vi "__List Drag Start Handler.vi"(8 "error in (no error)":errorcluster, 11 "MCListbox Refnum":refnum<vi>) -> (0 "error out":errorcluster, 2 "Discard Drag?":bool, 3 "Drag Data":T1(array[cluster]))   [LabVIEW 2011]
doc: "This VI decides if the drag operation is discarded on start (if the selected item is not a file in one of the listboxes).\nIn case the operation is allowed, it also created the necessary drag data."
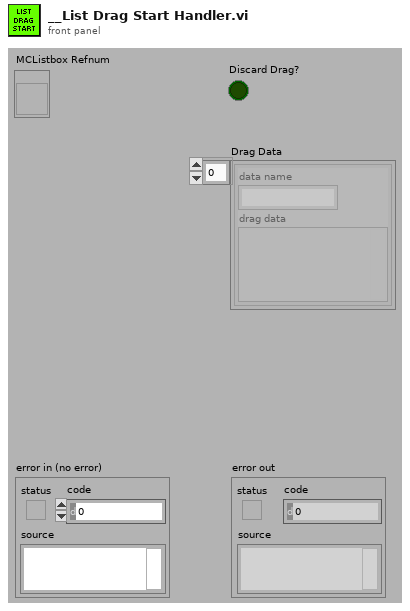
[diagram p1: front panel]
types:
  T1 = cluster{"data name":string, "drag data":variant}[]
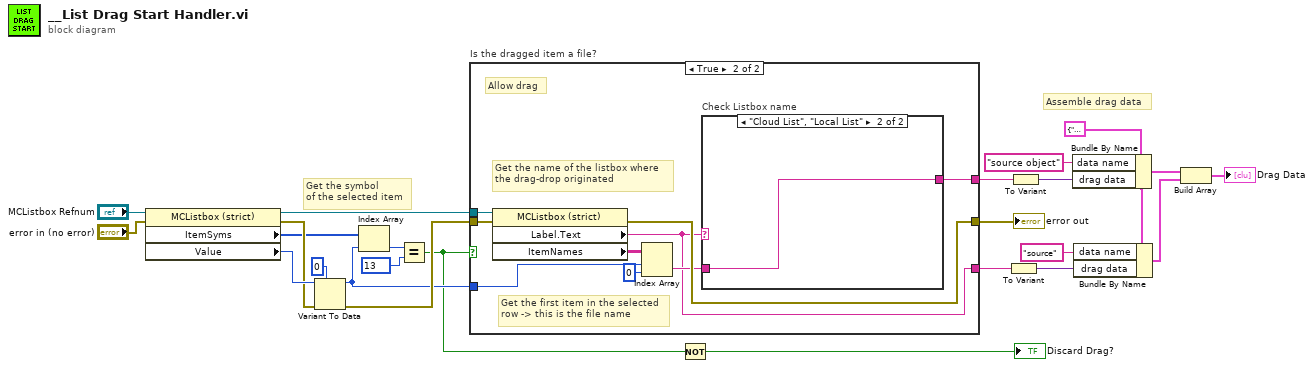
[diagram p0: block diagram]
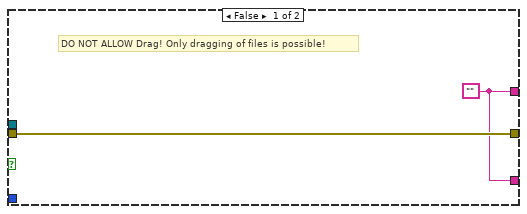
[diagram p2: hidden frame]
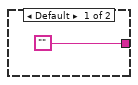
[diagram p3: hidden frame]
diagram:
  w6 = cluster{"data name":string, "drag data":variant} {"data name"="", "drag data"=variant}
  # "Assemble drag data"
  # "Get the symbol\nof the selected item"
  n1 = property on="Property Node" class="MCListbox (strict)"(reference="MCListbox Refnum", error in="error in (no error)") -> (reference out=w16:refnum<vi>, error out=w21:errorcluster, "ItemSyms"=w19:i32[], "Value"=w22:i32)
  n2 = Variant To Data(error in=w21, type=0, Variant=w22) -> (data=w14:i32, error out=w15:errorcluster)
  n3 = Index Array(array=w19, index=w14) -> (element=w18:i32)
  n4 = Equal?(x=w18, y=13) -> (x = y?=w2:bool)
  n5 = case "Is the dragged item a file?" shown="True" w2 {
    tunnel: w16 -> [_ w35]
    tunnel: w15 -> [w26 w34]
    tunnel: w14 -> [_ w32]
    tunnel: [w25 w30] -> w12
    tunnel: [w26 w29] -> w13
    tunnel: [w25 w27] -> w7
    frame False {
      w25 = ""
      # "DO NOT ALLOW Drag! Only dragging of files is possible!"
    }
    frame True {
      # "Get the first item in the selected\nrow -> this is the file name"
      # "Get the name of the listbox where\nthe drag-drop originated"
      # "Allow drag"
      n6 = property on="Property Node" class="MCListbox (strict)"(reference=w35, error in=w34) -> (error out=w29:errorcluster, "Label.Text"=w27:string, "ItemNames"=w33:string[][])  [unwired: 1 out]
      n7 = Index Array(array=w33, index (row)=w32, index (col)=0 ("disabled index (col)")) -> (element=w28:string)
      n8 = case "Check Listbox name" shown="\"Cloud List\", \"Local List\"" w27 {
        tunnel: w28 -> [_ w37]
        tunnel: ["" w37] -> w30
        frame Default {
        }
        frame "Cloud List", "Local List" {
        }
      }
    }
  }
  "error out" <- w13
  n9 = Not(x=w2) -> (.not. x?=→"Discard Drag?":bool)
  n10 = To Variant(anything=w7) -> (Variant=w4:variant)
  n11 = To Variant(anything=w12) -> (Variant=w11:variant)
  n12 = Bundle By Name(cluster=w6, "data name"="source object", "drag data"=w11) -> (w9:cluster{"data name":string, "drag data":variant})
  n13 = Bundle By Name(cluster=w6, "data name"="source", "drag data"=w4) -> (w3:cluster{"data name":string, "drag data":variant})
  n14 = Build Array(w9, w3) -> (→"Drag Data":T1)
